vi "Write targetPosition.vi"(8 "error in (no error)":errorcluster, 10 "targetPosition":dbl[](array[numeric]), 11 "Zone in":refnum<class "Zone.lvclass">) -> (0 "error out":errorcluster, 3 "Zone out":refnum<class "Zone.lvclass">)   [LabVIEW 2023, in "Zone.lvclass"]
uses:
  Zone.lvclass
  Zone.lvclass/Zone.ctl
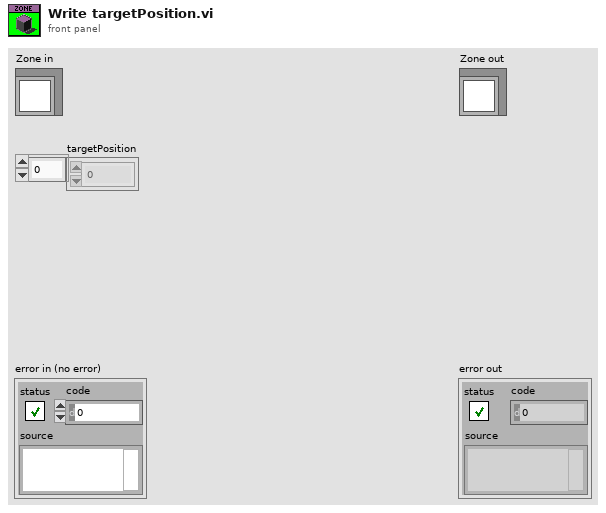
[diagram p1: front panel]
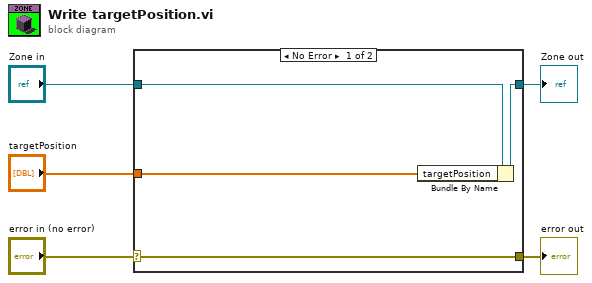
[diagram p0: block diagram]
diagram:
  n1 = case shown="No Error" "error in (no error)" {
    selector: "error in (no error)" -> [w9 w10]
    tunnel: [w9 w10] -> w4
    tunnel: [w7 w11] -> w2
    tunnel: "Zone in" -> [w8 w11]
    tunnel: "targetPosition" -> [w6 _]
    frame No Error {
      n2 = Bundle By Name(cluster=w8, "targetPosition"=w6) -> (w7:refnum<class "Zone.lvclass">)
    }
    frame Error {
    }
  }
  "error out" <- w4
  "Zone out" <- w2
